vi "Lift Control.vi"(8 "error in (no error)":errorcluster) -> ()   [LabVIEW 2014]
doc: "This VI runs in parallel to other tasks. It can contain as many user-defined periodic loops as you need. These can carry out PID or other sorts of timed response."
uses:
  Robot Global Data.vi
  <vilib>/addons/control/pid/pid.llb/PID (DBL).vi
  <vilib>/addons/control/pid/NI_PID_pid.lvlib
panel:
  in  "output range":cluster{"output high":dbl, "output low":dbl}={"output high"=0.7, "output low"=-0.7} {"output low" format="%.2f"; "output high" format="%.2f"}
  in  "PID gains":T1={"proportional gain (Kc)"=0.002, "integral time (Ti, min)"=0.0, "derivative time (Td, min)"=0.0} {"derivative time (Td, min)" format="%.3f"; "integral time (Ti, min)" format="%.3f"; "proportional gain (Kc)" format="%.3f"}
  in  "Level 5":dbl=4000.0
  in  "Level 4":dbl=3980.0
  in  "Level 3":dbl=2983.0
  in  "Level 2":dbl=2150.0
  in  "Level 1":dbl=958.0
  in  "Level G":dbl
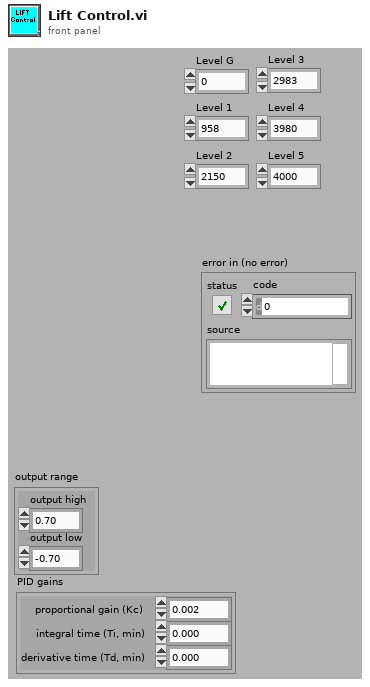
[diagram p1: front panel]
types:
  T1 = cluster{"proportional gain (Kc)":dbl, "integral time (Ti, min)":dbl, "derivative time (Td, min)":dbl}
  T2 = typedef "WPI_MotorControlDeviceRef.ctl" = cluster{"DeviceStatus":errorcluster, "Type":T3, "PWM":cluster{"Controller":T4, "PWM Channel":T5, "DeadBand":T6}, "CAN":cluster{"Device Number":u8, "Control Mode":T7, "Semaphore":T8, "Max Vout":dbl, "TalonSRX Control Mode":T9}, "Invert":bool, "TransformRef":T10, "InvTransformRef":T10}
  T3 = typedef "WPI_MotorControlType.ctl" = enum16{"PWM", "CAN", "CANTalonSRX"}
  T4 = typedef "FPGA_TypedefDigitalModule.ctl" = enum16{"Controller 1"}
  T5 = typedef "FPGA_DIOPWMChannel.ctl" = enum8{"PWM 0", "PWM 1", "PWM 2", "PWM 3", "PWM 4", "PWM 5", "PWM 6", "PWM 7", "PWM 8", "PWM 9", "PWM MXP 0", "PWM MXP 1", "PWM MXP 2", "PWM MXP 3", "PWM MXP 4", "PWM MXP 5", "PWM MXP 6", "PWM MXP 7", "PWM MXP 8", "PWM MXP 9", "Invalid"}
  T6 = typedef "WPI_PWMDeadband.ctl" = cluster{"Name":string, "maxPositivePwm":i32, "minPositivePwm":i32, "centerPwm":i32, "maxNegativePwm":i32, "minNegativePwm":i32, "angularRange":u16}
  T7 = typedef "WPI_CANJaguar_ControlMode.ctl" = enum8{"Percent VBus", "Current", "Speed", "Position", "Voltage"}
  T8 = typedef "Semaphore RefNum" = refnum<k1>
  T9 = typedef "WPI_CANTalonSRX_APIControlMode.ctl" = enum8{"Percent VBus", "Speed", "Position", "Slave", "Unchanged / Invalid"}
  T10 = typedef "WPI_PWMTransform_ConPane.ctl" = refnum<vi>
  T11 = typedef "WPI_EncoderDevRef.ctl" = cluster{"DevStatus":errorcluster, "EncoderIndex":T12, "CounterIndex":T13, "DistancePerCount":dbl, "Decoding Type":T14}
  T12 = typedef "FPGA_EncoderIdx.ctl" = enum8{"Enc 0", "Enc 1", "Enc 2", "Enc 3", "Enc 4", "Enc 5", "Enc 6", "Enc 7", "Invalid"}
  T13 = typedef "FPGA_CounterCtrSystemIndex.ctl" = enum8{"Ctr 0", "Ctr 1", "Ctr 2", "Ctr 3", "Ctr 4", "Ctr 5", "Ctr 6", "Ctr 7", "Invalid"}
  T14 = typedef "WPI_EncoderType.ctl" = enum16{"1x", "2x", "4x"}
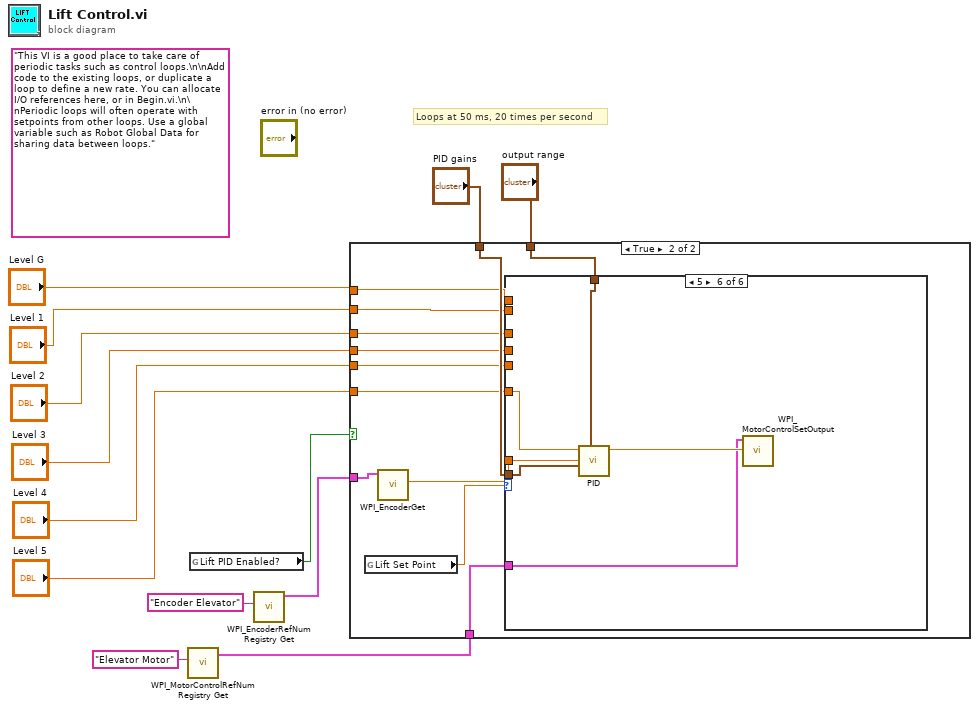
[diagram p0: block diagram]
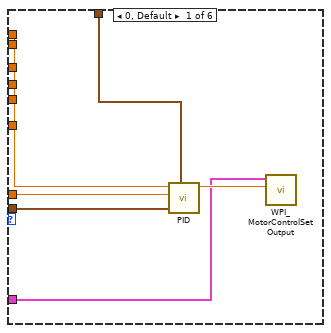
[diagram p3: hidden frame]
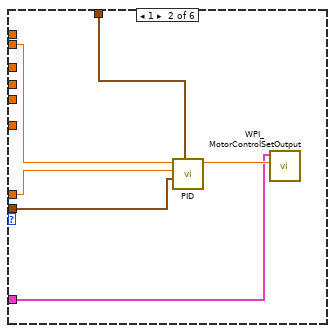
[diagram p4: hidden frame]
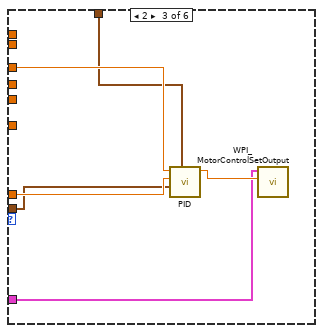
[diagram p5: hidden frame]
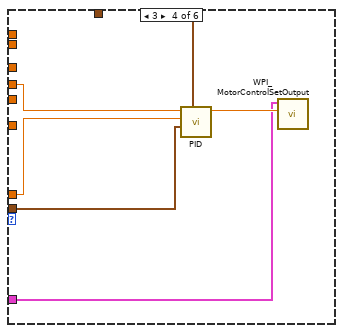
[diagram p6: hidden frame]
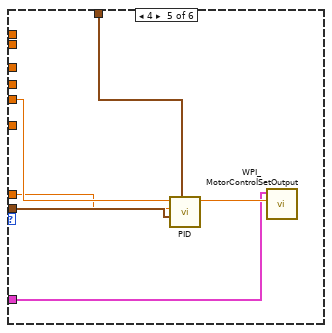
[diagram p7: hidden frame]
diagram:
  (unwired) "This VI is a good place to take care of periodic tasks such as control loops.\n\nAdd code to the existing loops, or duplicate a loop to define a new rate. You can allocate I/O references here, or in Begin.vi.\n\nPeriodic loops will often operate with setpoints from other loops. Use a global variable such as Robot Global Data for sharing data between loops."
  # "Loops at 50 ms, 20 times per second"
  n1 = call <vilib>:"WPI_MotorControlRefNum Registry Get.vi"("refnum name"="Elevator Motor") -> ("MotorControlDevRef"=w7:T2)  [unwired: 9 in, 1 out]
  n2 = global read "Robot Global Data.vi" "Lift PID Enabled?"() -> (w11:bool)
  n3 = call <vilib>:"WPI_EncoderRefNum Registry Get.vi"("refnum name"="Encoder Elevator") -> ("EncoderDevRef"=w1:T11)  [unwired: 9 in, 1 out]
  n4 = case shown="True" w11 {
    tunnel: "output range" -> [_ w15]
    tunnel: "PID gains" -> [_ w25]
    tunnel: w1 -> [_ w24]
    tunnel: "Level 1" -> [_ w22]
    tunnel: "Level 2" -> [_ w17]
    tunnel: "Level 3" -> [_ w21]
    tunnel: "Level 4" -> [_ w20]
    tunnel: "Level 5" -> [_ w19]
    tunnel: w7 -> [_ w18]
    tunnel: "Level G" -> [_ w14]
    frame False {
    }
    frame True {
      n5 = global read "Robot Global Data.vi" "Lift Set Point"() -> (w16:dbl)
      n6 = call <vilib>:"WPI_EncoderGet.vi"("EncoderDevRef"=w24) -> ("Distance"=w23:dbl)  [unwired: 5 in, 5 out]
      n7 = case shown="5" w16 {
        tunnel: w15 -> [w31 w37 w40 w46 w55 w58]
        tunnel: w25 -> [w30 w36 w41 w47 w54 w59]
        tunnel: w23 -> [w29 w35 w42 w48 w52 w60]
        tunnel: w14 -> [w28 _ _ _ _ _]
        tunnel: w22 -> [_ w34 _ _ _ _]
        tunnel: w17 -> [_ _ w43 _ _ _]
        tunnel: w21 -> [_ _ _ w49 _ _]
        tunnel: w20 -> [_ _ _ _ w53 _]
        tunnel: w19 -> [_ _ _ _ _ w61]
        tunnel: w18 -> [w26 w32 w38 w44 w50 w56]
        frame 0, Default {
          n8 = call-poly <vilib>:"PID.vi"("output range"=w31, "PID gains"=w30, "process variable"=w29, "setpoint"=w28) -> ("output"=w27:dbl)  [unwired: 6 in, 1 out]
          n9 = call <vilib>:"WPI_MotorControlSetOutput.vi"("Output"=w27, "MotorControlDevRef"=w26) -> ()  [unwired: 7 in, 3 out]
        }
        frame 1 {
          n10 = call-poly <vilib>:"PID.vi"("output range"=w37, "PID gains"=w36, "process variable"=w35, "setpoint"=w34) -> ("output"=w33:dbl)  [unwired: 6 in, 1 out]
          n11 = call <vilib>:"WPI_MotorControlSetOutput.vi"("Output"=w33, "MotorControlDevRef"=w32) -> ()  [unwired: 7 in, 3 out]
        }
        frame 2 {
          n12 = call-poly <vilib>:"PID.vi"("output range"=w40, "PID gains"=w41, "process variable"=w42, "setpoint"=w43) -> ("output"=w39:dbl)  [unwired: 6 in, 1 out]
          n13 = call <vilib>:"WPI_MotorControlSetOutput.vi"("Output"=w39, "MotorControlDevRef"=w38) -> ()  [unwired: 7 in, 3 out]
        }
        frame 3 {
          n14 = call-poly <vilib>:"PID.vi"("output range"=w46, "PID gains"=w47, "process variable"=w48, "setpoint"=w49) -> ("output"=w45:dbl)  [unwired: 6 in, 1 out]
          n15 = call <vilib>:"WPI_MotorControlSetOutput.vi"("Output"=w45, "MotorControlDevRef"=w44) -> ()  [unwired: 7 in, 3 out]
        }
        frame 4 {
          n16 = call-poly <vilib>:"PID.vi"("output range"=w55, "PID gains"=w54, "process variable"=w52, "setpoint"=w53) -> ("output"=w51:dbl)  [unwired: 6 in, 1 out]
          n17 = call <vilib>:"WPI_MotorControlSetOutput.vi"("Output"=w51, "MotorControlDevRef"=w50) -> ()  [unwired: 7 in, 3 out]
        }
        frame 5 {
          n18 = call-poly <vilib>:"PID.vi"("output range"=w58, "PID gains"=w59, "process variable"=w60, "setpoint"=w61) -> ("output"=w57:dbl)  [unwired: 6 in, 1 out]
          n19 = call <vilib>:"WPI_MotorControlSetOutput.vi"("Output"=w57, "MotorControlDevRef"=w56) -> ()  [unwired: 7 in, 3 out]
        }
      }
    }
  }
